vi "Testing Parsing 2D image.vi"(11 "2D Picture":picture) -> (2 "output array":u16[](array[numeric]), 3 "Background":T1 {"image" format="%.0x"})   [LabVIEW 2019]
uses:
  <vilib>/picture/picture.llb/imagedata.ctl
panel:
  out "Doodle":T1 {"image" format="%.0x"}
  out "new picture 2":picture
  out "new picture":picture
  out "image data":T1 {"image" format="%.0x"}
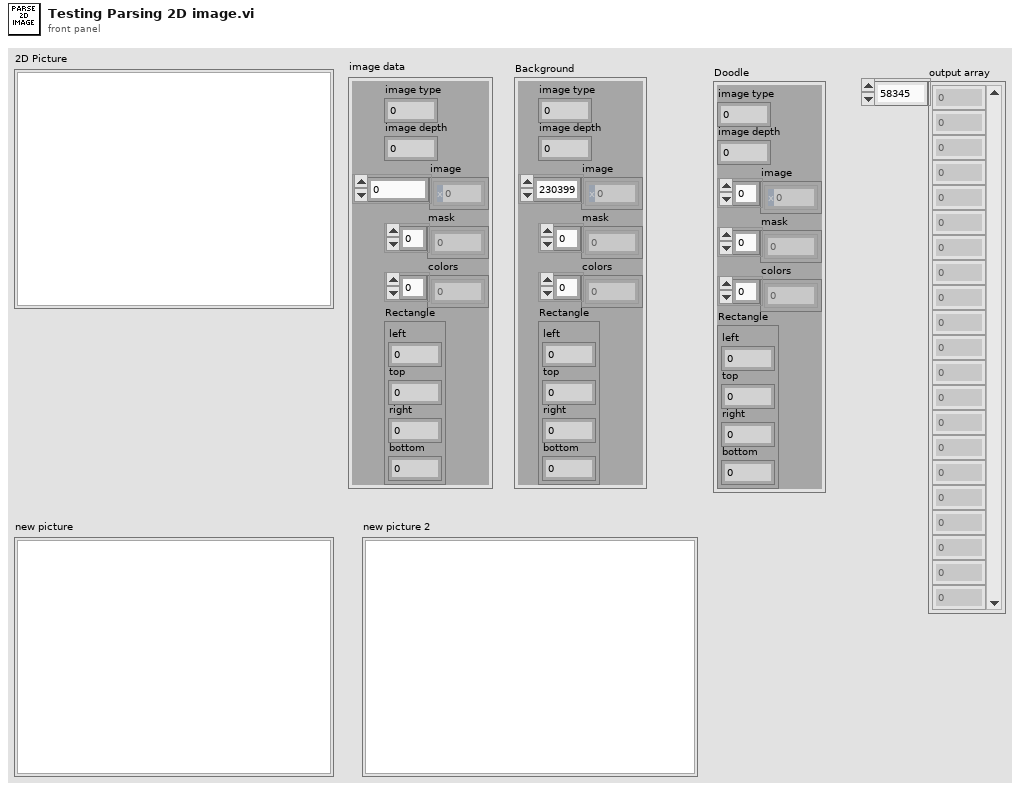
[diagram p1: front panel]
types:
  T1 = typedef "imagedata.ctl" = cluster{"image type":i32, "image depth":i32, "image":u8[], "mask":u8[], "colors":u32[], "Rectangle":cluster{"left":i16, "top":i16, "right":i16, "bottom":i16}}
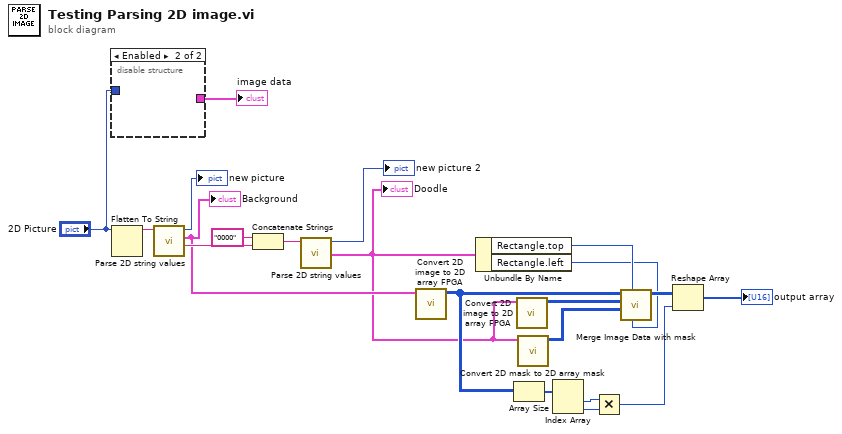
[diagram p0: block diagram]
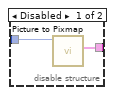
[diagram p2: hidden frame]
diagram:
  n1 = disable-structure shown="Enabled" {
    disable-tunnel: "2D Picture" -> [w23 _]
    disable-tunnel: [w22 _] -> w14
    frame Disabled {
      n2 = call <vilib>:"Picture to Pixmap.vi"("picture"=w23) -> ("image data"=w22:T1)  [unwired: 9 in, 1 out]
    }
    frame Enabled {
    }
  }
  "image data" <- w14
  n3 = Flatten To String(anything="2D Picture") -> (data string=w20:string)  [unwired: 3 in, 2 out]
  n4 = call "Parse 2D string values.vi"("data string in"=w20) -> ("substring 2"=w18:string, "image data"=w13:T1, "new picture"=→"new picture":picture)  [unwired: 8 in]
  "Background" <- w13
  n5 = Concatenate Strings("0000" ("string"), w18) -> (w17:string)
  n6 = call "Parse 2D string values.vi"("data string in"=w17) -> ("image data"=w3:T1, "new picture"=→"new picture 2":picture)  [unwired: 8 in, 1 out]
  "Doodle" <- w3
  n7 = call "Convert 2D image to 2D array FPGA.vi"("image data"=w13) -> ("data"=w5:u16[][])  [unwired: 10 in]
  n8 = Unbundle By Name(w3) -> ("Rectangle.top"=w2:i16, "Rectangle.left"=w1:i16)
  n9 = Array Size(array=w5) -> (size(s)=w9:i32[])
  n10 = call "Convert 2D image to 2D array FPGA.vi"("image data"=w3) -> ("data"=w4:u16[][])  [unwired: 10 in]
  n11 = call "Convert 2D mask to 2D array mask.vi"("image data"=w3) -> ("2D Mask"=w11:u8[][])  [unwired: 10 in]
  n12 = Index Array(array=w9) -> (element #1=w8:i32, element #2=w7:i32)  [unwired: 2 in]
  n13 = Multiply(x=w8, y=w7) -> (x*y=w6:i32)
  n14 = call "Merge Image Data with mask.vi"("Col"=w1, "Row"=w2, "Mask"=w11, "Image Data 2"=w4, "Image Data 1"=w5) -> ("Merged Data"=w10:u16[][])  [unwired: 6 in]
  n15 = Reshape Array(w10, w6) -> (→"output array":u16[])
